vi "VCS Get Dc Motor Parameter Ex.vi"(0 "axis in":cluster{"keyHandle":u32, "nodeId":u16}={"keyHandle"=0, "nodeId"=1}, 11 "error in (no error)":errorcluster) -> (4 "axis out":cluster{"keyHandle":u32, "nodeId":u16}={"keyHandle"=0, "nodeId"=1}, 8 "DC motor parameter ex":T1, 15 "error out":errorcluster)   [LabVIEW 2017, in "maxonEPOS.lvlib"]
doc: "With function <B>VCS_GetDcMotorParameter</B> it is possible to read all DC motor parameters."
uses:
  Examples/maxonEPOS.lvlib
  Resources/EposCmd.dll
  SSI_Tool/InstrumentsInterfaces/Motordriver/maxon EPOS/Resources/EposCmd64.dll
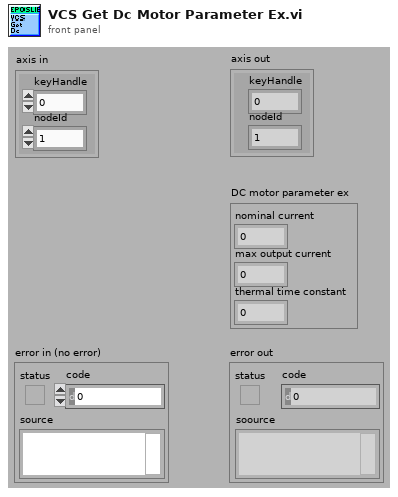
[diagram p1: front panel]
types:
  T1 = cluster{"nominal current":u32, "max output current":u32, "thermal time constant":u16}
  T2 = cluster{"pNominalCurrent":u16, "pMaxOutputCurrent":u16, "pThermalTimeConstant":u16}
  T3 = cluster{"pNominalCurrent":u32, "pMaxOutputCurrent":u32, "pThermalTimeConstant":u16}
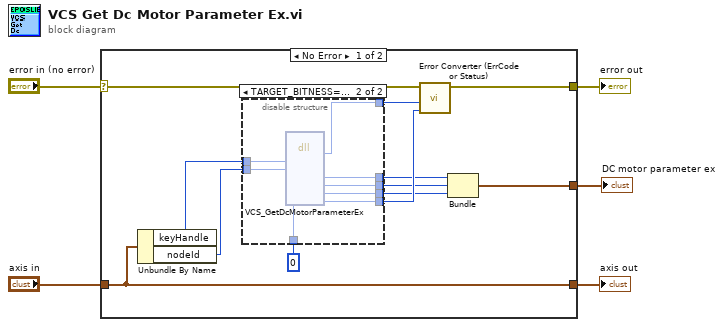
[diagram p0: block diagram]
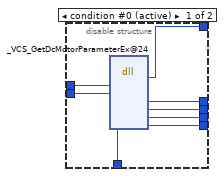
[diagram p2: hidden frame]
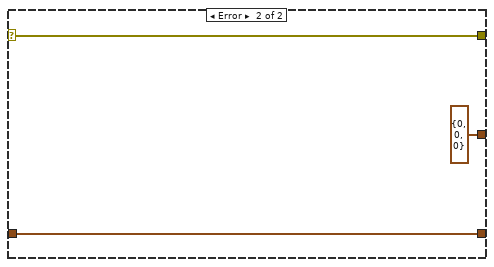
[diagram p3: hidden frame]
diagram:
  n1 = case shown="No Error" "error in (no error)" {
    selector: "error in (no error)" -> [w15 w35]
    tunnel: "axis in" -> [w17 w36]
    tunnel: [w17 w36] -> w4
    tunnel: [w16 w35] -> w3
    tunnel: [w6 T2 {"pNominalCurrent"=0, "pMaxOutputCurrent"=0, "pThermalTimeConstant"=0}] -> w1
    frame No Error {
      n2 = Unbundle By Name(w17) -> ("keyHandle"=w12:u32, "nodeId"=w13:u16)
      n3 = disable-structure shown="TARGET_BITNESS==64" {
        disable-tunnel: u32 0 ("pErrorCode") -> [w25 w33]
        disable-tunnel: w13 -> [w24 w32]
        disable-tunnel: w12 -> [w23 w31]
        disable-tunnel: [w22 w30] -> w11
        disable-tunnel: [w21 w29] -> w10
        disable-tunnel: [w20 w28] -> w9
        disable-tunnel: [w19 w27] -> w8
        disable-tunnel: [w18 w26] -> w7
        frame condition #0 (active) {
          n4 = dll-call lib="C:/workspace/project/scancon/sw/SSI_Tool/InstrumentsInterfaces/Motordriver/maxon EPOS/Resources/EposCmd.*" fn="_VCS_GetDcMotorParameterEx@24" ("EposCmd.dll:_VCS_GetDcMotorParameter@24")("KeyHandle"=w23, "NodeId"=w24, "pErrorCode"=w25) -> ("Rückgabetyp"=w22:i32, "pNominalCurrent"=w20:u32, "pMaxOutputCurrent"=w19:u32, "pThermalTimeConstant"=w18:u16, "pErrorCode"=w21:u32)  [unwired: 8 in, 2 out]
        }
        frame condition #1 {
          n5 = dll-call lib="C:/Sources/LabView/maxon EPOS/Resources/EposCmd64.*" fn="VCS_GetDcMotorParameterEx" ("EposCmd.dll:_VCS_GetDcMotorParameter@24")("KeyHandle"=w31, "NodeId"=w32, "pErrorCode"=w33) -> ("Rückgabetyp"=w30:i32, "pNominalCurrent"=w28:u32, "pMaxOutputCurrent"=w27:u32, "pThermalTimeConstant"=w26:u16, "pErrorCode"=w29:u32)  [unwired: 8 in, 2 out]
        }
      }
      n6 = call "Error Converter (ErrCode or Status).vi"("error code"=w10, "return type"=w11, "error in (no error)"=w15) -> ("error out"=w16:errorcluster)  [unwired: 7 in]
      n7 = Bundle("pNominalCurrent"=w9, "pMaxOutputCurrent"=w8, "pThermalTimeConstant"=w7) -> (w6:T3)  [unwired: 1 in]
    }
    frame Error {
    }
  }
  "error out" <- w3
  "axis out" <- w4
  "DC motor parameter ex" <- w1
